vi "Update_FI.vi"(7 "Reset":bool=TRUE, 8 "input valid":bool=TRUE, 10 "Fi_delta":fxp<+/-,32,4>, 11 "Fi_start":fxp<+/-,32,4>) -> (0 "output valid":bool, 3 "Fi out":fxp<+/-,32,4>)   [LabVIEW 2013]
doc: "Increases Fi with Fi_delta. Also wraps Fi to the range [0, 2*Pi]"
uses:
  <vilib>/rvi/FXPMathLib/FxpAdd/XNode/nifxpmath_Add.xnode
  <vilib>/rvi/FXPMathLib/sim/FxpSim.dll
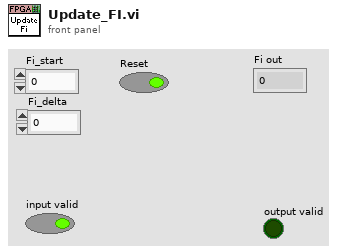
[diagram p1: front panel]
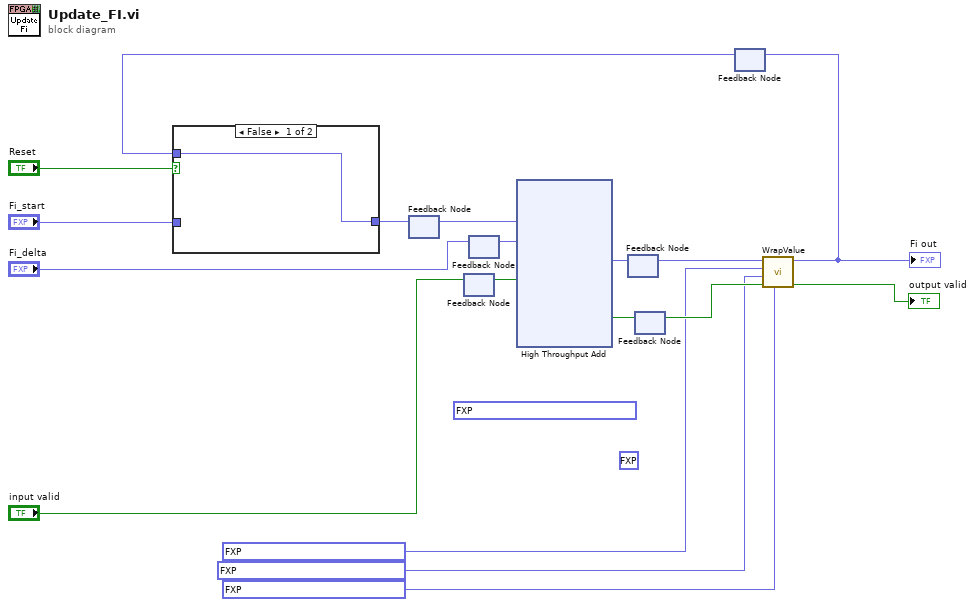
[diagram p0: block diagram]
diagram:
  (unwired) fxp<+/-,32,4> 0.0 ("wrap_max")
  (unwired) fxp<+/-,32,4> 6.2831853069365025 ("wrap_max")
  n1 = feedback #1() -> (w13:fxp<+/-,32,4>)  [unwired: 1 in]
  n2 = feedback #2() -> (w10:bool)  [unwired: 1 in]
  n3 = feedback-in #2("input valid") -> ()
  n4 = feedback #3() -> (w12:fxp<+/-,32,4>)  [unwired: 1 in]
  n5 = feedback-in #3("Fi_delta") -> ()
  n6 = xnode "High Throughput Add"("x"=w13, "y"=w12, "input valid"=w10) -> ("x+y"=w18:fxp<+/-,32,4>, "output valid"=w15:bool)  [unwired: 1 in, 1 out]
  n7 = feedback-in #4(w18) -> ()
  n8 = feedback #4() -> (w9:fxp<+/-,32,4>)  [unwired: 1 in]
  n9 = feedback #5() -> (w8:bool)  [unwired: 1 in]
  n10 = feedback-in #5(w15) -> ()
  n11 = feedback #6() -> (w7:fxp<+/-,32,4>)  [unwired: 1 in]
  n12 = case shown="False" "Reset" {
    tunnel: "Fi_start" -> [_ w20]
    tunnel: [w19 w20] -> w14
    tunnel: w7 -> [w19 _]
    frame False {
    }
    frame True {
    }
  }
  n13 = feedback-in #1(w14) -> ()
  n14 = call "WrapValue.vi"("wrap_range"=fxp<+/-,32,4> 6.2831853069365025 ("wrap_max"), "Input valid"=w8, "wrap_min"=fxp<+/-,32,4> -3.1415926553308964 ("wrap_max"), "wrap_max"=fxp<+/-,32,4> 3.1415926553308964, "x_in"=w9) -> ("output valid"=→"output valid":bool, "x_out"=w4:fxp<+/-,32,4>)  [unwired: 5 in]
  "Fi out" <- w4
  n15 = feedback-in #6(w4) -> ()
